vi "Variant Cluster to JSON.vi"(8 "error in":errorcluster, 11 "Variant":variant) -> (0 "error out":errorcluster, 3 "String":string)   [LabVIEW 2011]
uses:
  <userlib>/_OpenG.lib/lvdata/lvdata.llb/Type Descriptor Enumeration__ogtk.ctl
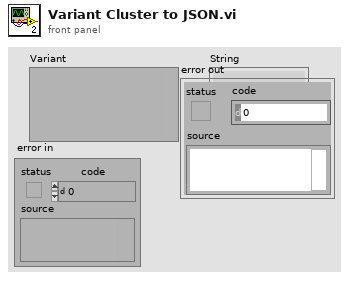
[diagram p1: front panel]
types:
  T1 = typedef "Type Descriptor Enumeration__ogtk.ctl" = enum8{"<Null>", "I8", "I16", "I32", "I64", "U8", "U16", "U32", "U64", "SGL", "DBL", "EXT", "CSG", "CDB", "CXT", "0x0F", "0x10", "0x11", "0x12", "0x13", "0x14", "Enum U8", "Enum U16", "Enum U32", "Enum U64", "SGL PQ", "DBL PQ", "EXT PQ", "CSG PQ", "CDB PQ", "CXT PQ", "0x1F", "0x20", "Boolean", "0x22", "0x23", "0x24", "0x25", "0x26", "0x27", "0x28", "0x29", "0x2A", "0x2B", "0x2C", "0x2D", "0x2E", "0x2F", "String", "0x31", "Path", "Pict", "0x34", "0x35", "0x36", "DAQ", "0x38", "0x39", "0x3A", "0x3B", "0x3C", "0x3D", "0x3E", "0x3F", "Array", "0x41", "0x42", "0x43", "0x44", "0x45", "0x46", "0x47", "0x48", "0x49", "0x4A", "0x4B", "0x4C", "0x4D", "0x4E", "0x4F", "Cluster", "0x51", "0x52", "Variant", "Waveform", "0x55", "0x56", "0x57", "0x58", "0x59", "0x5A", "0x5B", "0x5C", "0x5D", "0x5E", "0x5F", "0x60", "0x61", "0x62", "0x63", "0x64", "0x65", "0x66", "0x67", "0x68", "0x69", "0x6A", "0x6B", "0x6C", "0x6D", "0x6E", "0x6F", "Refnum"}
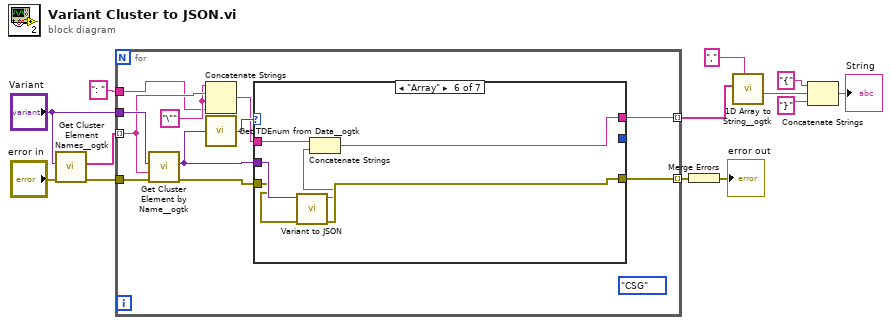
[diagram p0: block diagram]
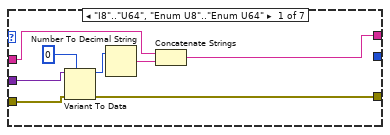
[diagram p2: hidden frame]
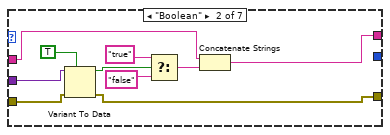
[diagram p3: hidden frame]
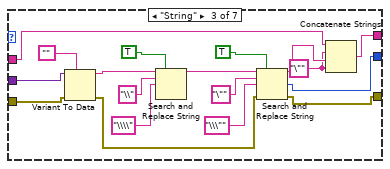
[diagram p4: hidden frame]
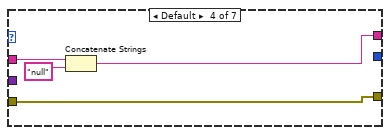
[diagram p5: hidden frame]
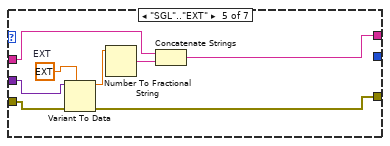
[diagram p6: hidden frame]
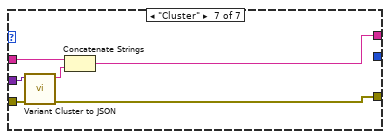
[diagram p7: hidden frame]
diagram:
  n1 = call <userlib>:"Get Cluster Element Names__ogtk.vi"("error in (no error)"="error in", "Cluster"="Variant") -> ("error out"=w3:errorcluster, "Element Names"=w5:string[])  [unwired: 8 in]
  n2 = for {
    tunnel: w5 -> [w19] mode=indexing
    tunnel: "Variant" -> [w24]
    tunnel: ": " ("string") -> [w17]
    tunnel: [w21] -> w8 mode=indexing
    tunnel: w3 -> [w16]
    tunnel: [w14] -> w2 mode=indexing
    (unwired) Type_Descriptor_Enumeration__ogtk."CSG" ("Type Descriptor Enumeration")
    w18 = "\"" ("string")
    n3 = call <userlib>:"Get Cluster Element by Name__ogtk.vi"("error in (no error)"=w16, "Element Name"=w19, "Cluster"=w24) -> ("error out"=w15:errorcluster, "VElement"=w23:variant)  [unwired: 6 in, 1 out]
    n4 = Concatenate Strings(w18, w19, w18, w17) -> (w20:string)
    n5 = call <userlib>:"Get TDEnum from Data__ogtk.vi"("Data"=w23) -> ("Type Descriptor Enumeration"=w22:T1)  [unwired: 4 in]
    n6 = case shown="\"Array\"" w22 {
      tunnel: w23 -> [w32 w41 w60 _ w72 w76 w84]
      tunnel: w20 -> [w29 w42 w58 w64 w69 w78 w83]
      tunnel: [w28 w36 w57 w62 w68 w77 w82] -> w21
      tunnel: [_ _ w51 _ _ _ _] -> _
      tunnel: w15 -> [w26 w34 w50 w61 w66 w75 w80]
      tunnel: [w25 w33 w48 w61 w65 w74 w79] -> w14
      frame "I8".."U64", "Enum U8".."Enum U64" {
        n7 = Variant To Data(error in=w26, type=i64 0, Variant=w32) -> (data=w30:i64, error out=w25:errorcluster)
        n8 = Number To Decimal String(number=w30) -> (decimal integer string=w27:string)  [unwired: 1 in]
        n9 = Concatenate Strings(w29, w27) -> (w28:string)
      }
      frame "Boolean" {
        n10 = Variant To Data(error in=w34, type=TRUE, Variant=w41) -> (data=w39:bool, error out=w33:errorcluster)
        n11 = Select(t="true" ("string"), s=w39, f="false" ("string")) -> (s? t:f=w35:string)
        n12 = Concatenate Strings(w42, w35) -> (w36:string)
      }
      frame "String" {
        w52 = "\"" ("string")
        n13 = Variant To Data(error in=w50, type="", Variant=w60) -> (data=w47:string, error out=w49:errorcluster)
        n14 = Search and Replace String(replace all?=TRUE ("replace all? (F)"), input string=w47, search string="\\", replace string="\\\\" ("replace string (\"\")")) -> (result string=w43:string)  [unwired: 4 in, 3 out]
        n15 = Search and Replace String(replace all?=TRUE ("replace all? (F)"), input string=w43, search string="\"", replace string="\\\"" ("replace string (\"\")"), error in=w49) -> (result string=w54:string, number of replacements=w51:i32, error out=w48:errorcluster)  [unwired: 3 in, 1 out]
        n16 = Concatenate Strings(w58, w52, w54, w52) -> (w57:string)
      }
      frame Default {
        n17 = Concatenate Strings(w64, "null" ("string")) -> (w62:string)
      }
      frame "SGL".."EXT" {
        w71 = ext 0.0  # EXT
        n18 = Variant To Data(error in=w66, type=w71, Variant=w72) -> (data=w70:ext, error out=w65:errorcluster)
        n19 = Number To Fractional String(number=w70) -> (F-format string=w67:string)  [unwired: 3 in]
        n20 = Concatenate Strings(w69, w67) -> (w68:string)
      }
      frame "Array" {
        n21 = call "Variant to JSON.vi"("error in"=w75, "variant"=w76) -> ("error out"=w74:errorcluster, "concatenated string"=w73:string)  [unwired: 8 in]
        n22 = Concatenate Strings(w78, w73) -> (w77:string)
      }
      frame "Cluster" {
        n23 = call "Variant Cluster to JSON.vi"("error in"=w80, "Variant"=w84) -> ("error out"=w79:errorcluster, "String"=w81:string)  [unwired: 8 in]
        n24 = Concatenate Strings(w83, w81) -> (w82:string)
      }
    }
  }
  n25 = Merge Errors(w2) -> (→"error out":errorcluster)
  n26 = call <userlib>:"1D Array to String__ogtk.vi"("delimiter (Tab)"=",", "Array of Strings"=w8) -> ("delimited string"=w9:string)  [unwired: 9 in]
  n27 = Concatenate Strings("{" ("string"), w9, "}" ("string")) -> (→"String":string)
